vi "Execute.vi"(8 "error in (no error)":errorcluster caption="Fehler (Eingang, kein Fehler)", 11 "ApllicationLoadAndConfigurationClass Eingang":refnum<class "ApllicationLoadAndConfigurationClass.lvclass"> caption="DNL_LabVIEW Object in") -> (0 "error out":errorcluster caption="Fehler (Ausgang)", 3 "ApllicationLoadAndConfigurationClass Ausgang":refnum<class "ApllicationLoadAndConfigurationClass.lvclass"> caption="DNL_LabVIEW Object out")   [LabVIEW 2013, in "ApllicationLoadAndConfigurationClass.lvclass"]
uses:
  ApllicationLoadAndConfigurationClass.lvclass
panel:
  in  "WhereIGetMyInformation":string
  in  "WhoIAm":string
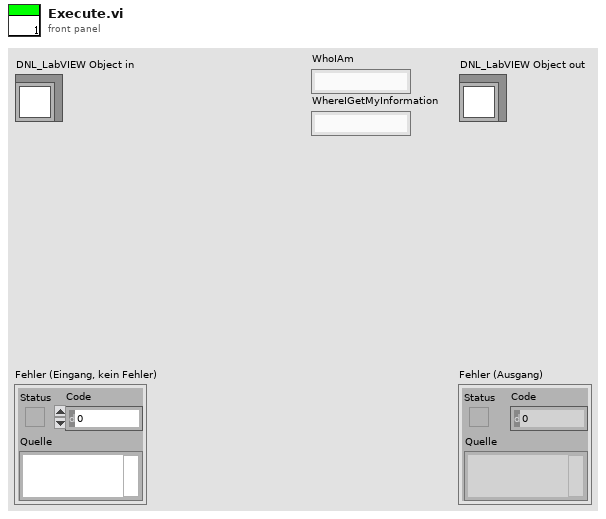
[diagram p1: front panel]
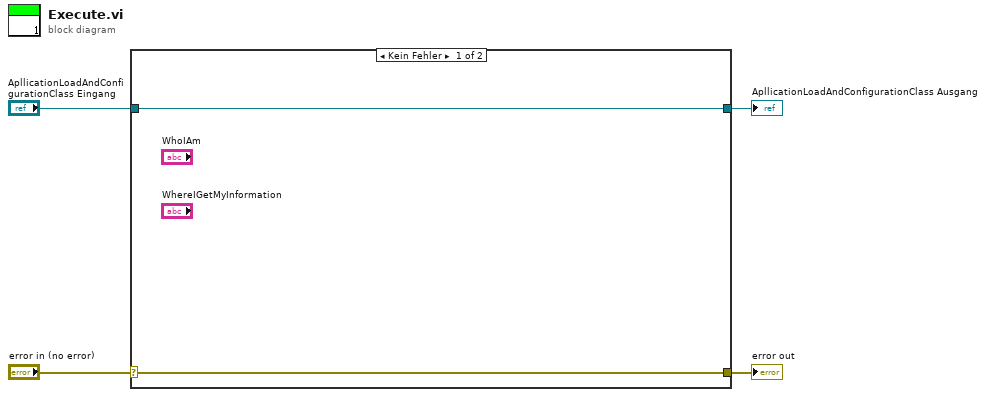
[diagram p0: block diagram]
diagram:
  n1 = case shown="Kein Fehler" "error in (no error)" {
    selector: "error in (no error)" -> [w6 w8]
    tunnel: [w6 w8] -> w3
    tunnel: [w5 w7] -> w1
    tunnel: "ApllicationLoadAndConfigurationClass Eingang" -> [w5 w7]
    frame No Error {
    }
    frame Error {
    }
  }
  "error out" <- w3
  "ApllicationLoadAndConfigurationClass Ausgang" <- w1
